vi "AE Camera Coral Image.vi"(7 "Update":bool, 11 "Ball Image in":T1(plugin-control)=refnum) -> (3 "Ball Image out":T1(plugin-control))   [LabVIEW 2025]
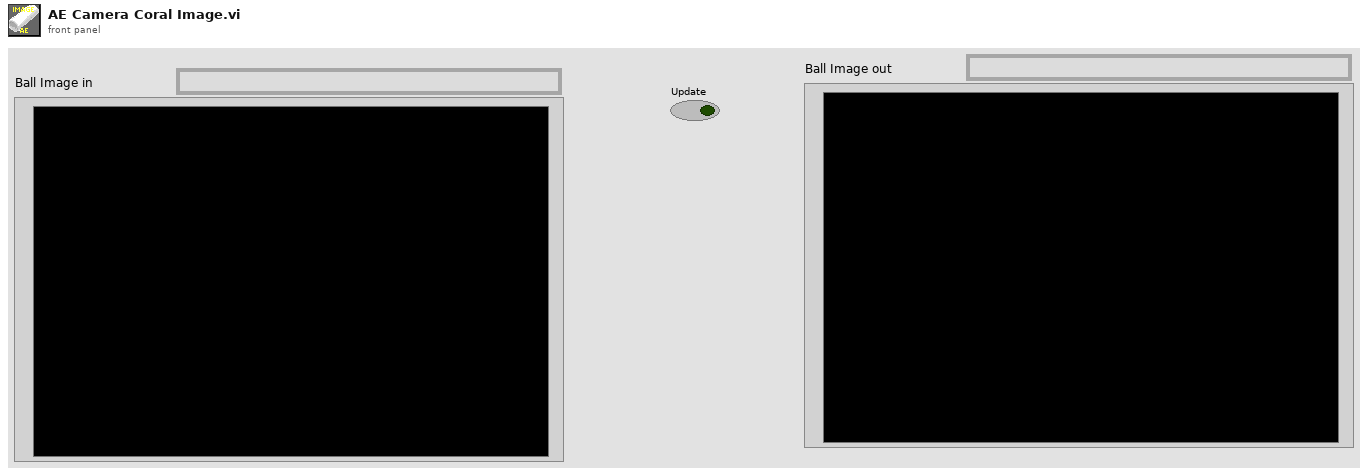
[diagram p1: front panel]
types:
  T1 = typedef "IMAQ Image.ctl" = refnum<image>
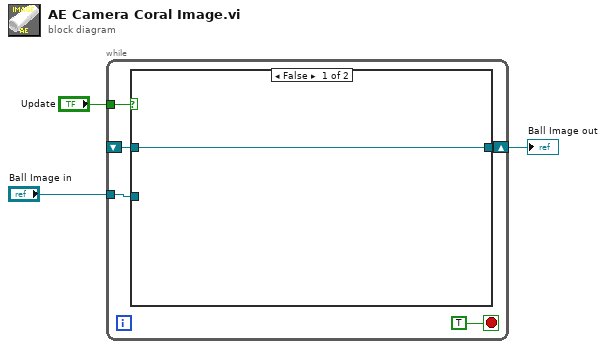
[diagram p0: block diagram]
diagram:
  n1 = while {
    tunnel: "Update" -> [w8]
    tunnel: "Ball Image in" -> [w7]
    shift-right: [w6] -> w1
    shift-left: _ -> [w5]
    stop <- TRUE stop-if-true
    n2 = case shown="False" w8 {
      tunnel: w7 -> [_ w10]
      tunnel: [w9 w10] -> w6
      tunnel: w5 -> [w9 _]
      frame False {
      }
      frame True {
      }
    }
  }
  "Ball Image out" <- w1
